vi "Create ToolStripProgressBar.vi"(8 "error in (no error)":errorcluster caption="错误输入（无错误）", 11 "name":string) -> (0 "error out":errorcluster caption="错误输出", 3 "ToolStripProgressBar 输出":refnum<class "ToolStripProgressBar.lvclass"> caption="DNL_LabVIEW Object out")   [LabVIEW 2013, in "ToolStripProgressBar.lvclass"]
uses:
  ToolStripProgressBar.lvclass
  System.Windows.Forms
  ToolStripProgressBar.lvclass/ToolStripProgressBar.ctl
panel:
  in  "ToolStripProgressBar 输入":refnum<class "ToolStripProgressBar.lvclass"> caption="DNL_LabVIEW Object in"
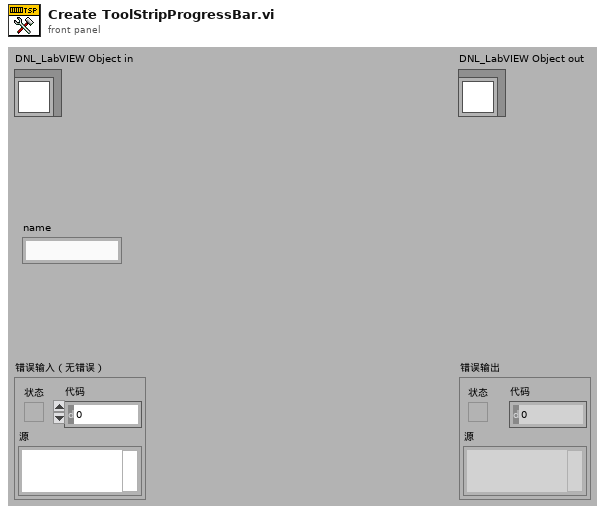
[diagram p1: front panel]
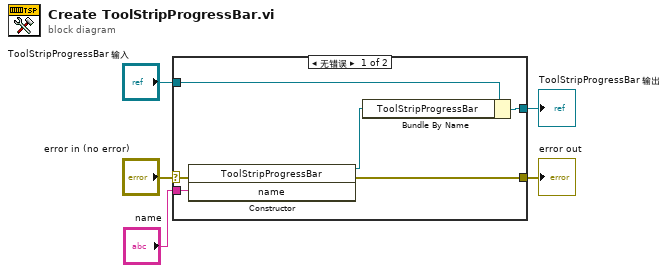
[diagram p0: block diagram]
diagram:
  n1 = case shown="无错误" "error in (no error)" {
    selector: "error in (no error)" -> [w8 w13]
    tunnel: [w6 w13] -> w4
    tunnel: [w9 w12] -> w2
    tunnel: "ToolStripProgressBar 输入" -> [w11 w12]
    tunnel: "name" -> [w7 _]
    frame No Error {
      n2 = constructor class="ToolStripProgressBar"(error in=w8, "name"=w7) -> (reference out=w10:refnum<k24>, error out=w6:errorcluster)  [unwired: 2 in, 2 out]
      n3 = Bundle By Name(cluster=w11, "ToolStripProgressBar"=w10) -> (w9:refnum<class "ToolStripProgressBar.lvclass">)
    }
    frame Error {
    }
  }
  "error out" <- w4
  "ToolStripProgressBar 输出" <- w2
